vi "GwyddionFileHeader.vi"(8 "error in":errorcluster, 11 "Filename":string) -> (0 "error out":errorcluster)   [LabVIEW 2016]
uses:
  controls/Enum.ctl
  libgwyscan-1.2-labview2015-win32/libgwyscan.lvlib
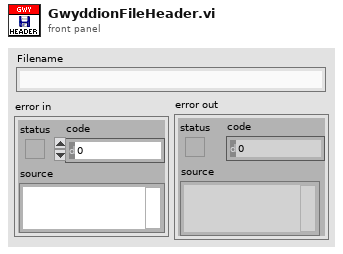
[diagram p1: front panel]
types:
  T1 = typedef "Enum.ctl" = enum16{"Init", "Read", "Write"}
  T2 = cluster{"calibName":string[], "calibParameters":cluster{"Sensitivity":cluster{"Sens X":dbl, "Sens Y":dbl, "Sens Z":dbl}, "Range":cluster{"Range X":dbl, "Range Y":dbl, "Range Z":dbl}, "HV gain":cluster{"HV gain X":dbl, "HV gain Y":dbl, "HV gain Z":dbl}}[], "calibIndex":i32}
  T3 = cluster{"Sensitivity":cluster{"Sens X":dbl, "Sens Y":dbl, "Sens Z":dbl}, "Range":cluster{"Range X":dbl, "Range Y":dbl, "Range Z":dbl}, "HV gain":cluster{"HV gain X":dbl, "HV gain Y":dbl, "HV gain Z":dbl}}[]
  T4 = cluster{"channelsToSaveOut":u8[], "Units":string[], "Saving":cluster{"Fwd":i32[], "Bwd":i32[]}, "x":i32[]}
  T5 = cluster{"Units":string[], "Offsets":dbl[], "Calibrations":dbl[]}
  T6 = cluster{"Sensitivity":cluster{"Sens X":dbl, "Sens Y":dbl, "Sens Z":dbl}, "Range":cluster{"Range X":dbl, "Range Y":dbl, "Range Z":dbl}, "HV gain":cluster{"HV gain X":dbl, "HV gain Y":dbl, "HV gain Z":dbl}}
  T7 = cluster{"Width":dbl, "Height":dbl, "X Offset":dbl, "Y Offset":dbl, "Angle":dbl, "Pixels/Line":u16, "Lines":u16, "Time/Line":dbl, "Scan Rate":dbl}
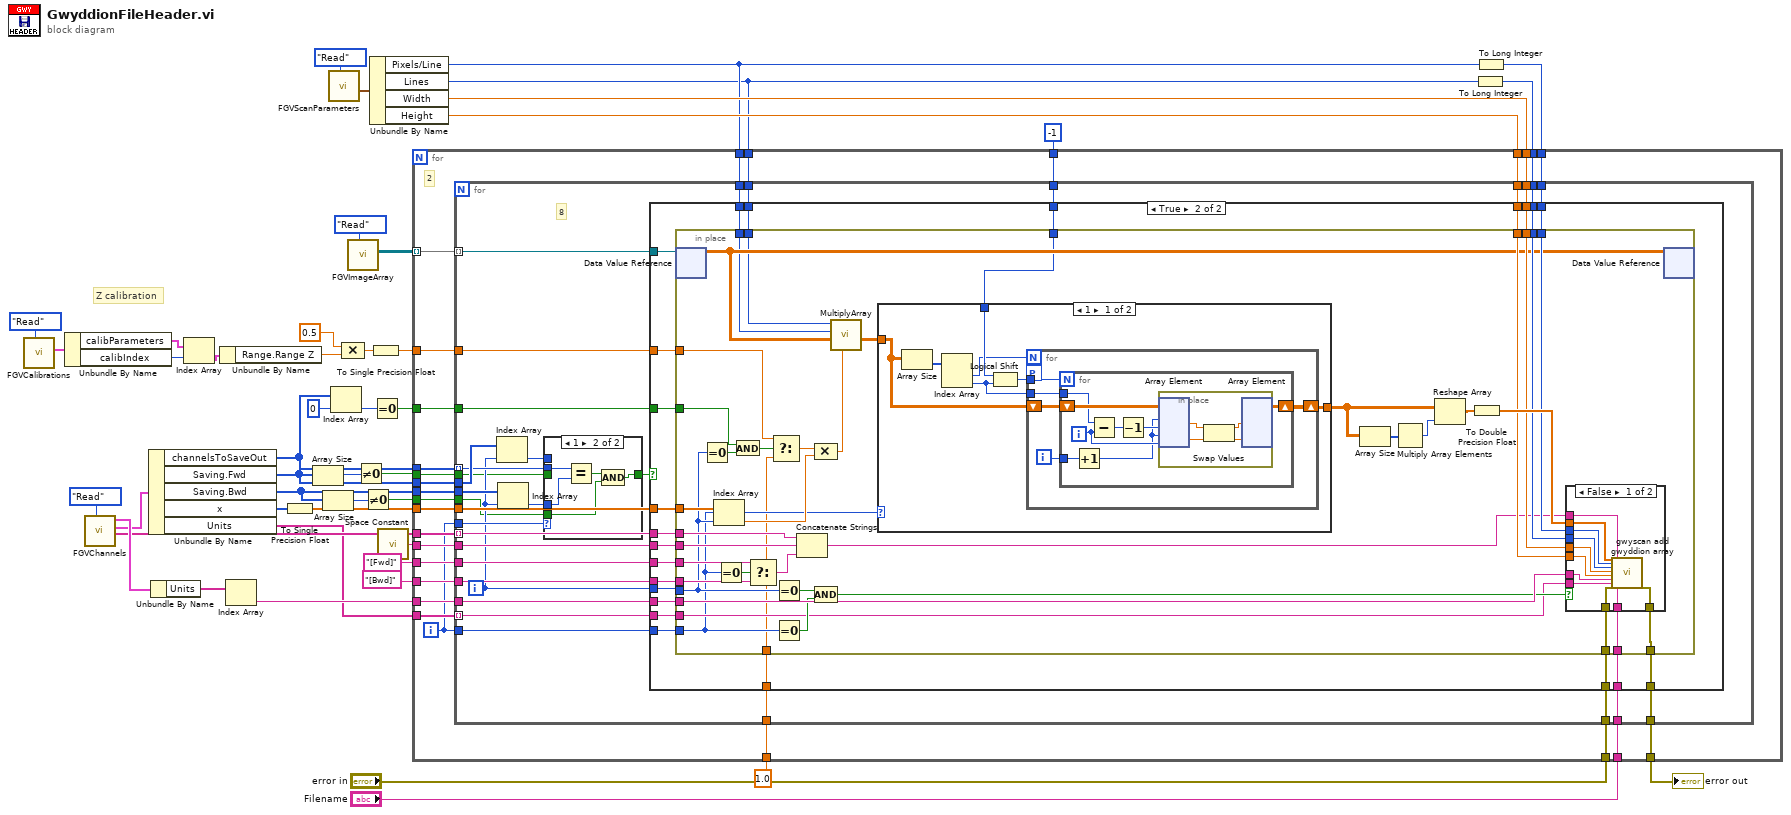
[diagram p0: block diagram]
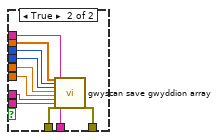
[diagram p3: hidden frame]
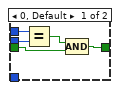
[diagram p5: hidden frame]
diagram:
  # "Z calibration"
  n1 = call "FGVCalibrations.vi"("Enum"=Enum."Read") -> ("calibOut"=w44:T2)  [unwired: 9 in, 1 out]
  n2 = Unbundle By Name(w44) -> ("calibParameters"=w43:T3, "calibIndex"=w42:i32)
  n3 = call "FGVChannels.vi"("Enum"=Enum."Read") -> ("channelsNamesOut"=w26:string[], "SavingChoiceOut"=w12:T4, "XYZ Units/Cal/Offset Out"=w38:T5)  [unwired: 6 in, 2 out]
  n4 = Unbundle By Name(w12) -> ("channelsToSaveOut"=w8:u8[], "Saving.Fwd"=w6:i32[], "Saving.Bwd"=w7:i32[], "x"=w11:i32[], "Units"=w9:string[])
  n5 = Unbundle By Name(w38) -> ("Units"=w35:string[])
  n6 = Index Array(array=w43, index=w42) -> (element=w41:T6)
  n7 = Unbundle By Name(w41) -> ("Range.Range Z"=w40:dbl)
  n8 = Index Array(array=w35) -> (element=w30:string)  [unwired: 1 in]
  n9 = To Single Precision Float(number=w11) -> (single precision float=w10:sgl[])
  n10 = Array Size(array=w6) -> (size(s)=w4:i32)
  n11 = Array Size(array=w7) -> (size(s)=w5:i32)
  n12 = call "FGVScanParameters.vi"("Enum"=Enum."Read") -> ("Scan Parameters Out"=w31:T7)  [unwired: 9 in, 1 out]
  n13 = Index Array(array=w8, index=0) -> (element=w14:u8)
  n14 = Compound Arithmetic op=MULTIPLY(0.5 ("x"), w40) -> (w37:dbl)
  n15 = call "FGVImageArray.vi"("Enum"=Enum."Read") -> ("ImageRefOut"=w34:refnum<data-value>[][])  [unwired: 9 in, 1 out]
  n16 = Not Equal To 0?(x=w4) -> (x != 0?=w3:bool)
  n17 = Not Equal To 0?(x=w5) -> (x != 0?=w2:bool)
  n18 = Unbundle By Name(w31) -> ("Pixels/Line"=w18:u16, "Lines"=w17:u16, "Width"=w20:dbl, "Height"=w19:dbl)
  n19 = To Single Precision Float(number=w37) -> (single precision float=w33:sgl)
  n20 = Equal To 0?(x=w14) -> (x = 0?=w13:bool)
  n21 = call <vilib>:"Space Constant.vi"() -> ("String"=w27:string)
  n22 = To Long Integer(number=w17) -> (32bit integer=w24:i32)
  n23 = To Long Integer(number=w18) -> (32bit integer=w25:i32)
  n24 = for {
    tunnel: w34 -> [w73] mode=indexing
    tunnel: w33 -> [w72]
    tunnel: w30 -> [w71]
    tunnel: "[Bwd]" -> [w70]
    tunnel: "[Fwd]" -> [w69]
    tunnel: w27 -> [w68]
    tunnel: w26 -> [w67]
    tunnel: w9 -> [w66]
    tunnel: w25 -> [w65]
    tunnel: w24 -> [w64]
    tunnel: w20 -> [w63]
    tunnel: w19 -> [w62]
    tunnel: "Filename" -> [w61]
    tunnel: "error in" -> [w60]
    tunnel: [w59] -> w21
    tunnel: w18 -> [w58]
    tunnel: w17 -> [w57]
    tunnel: i16 -1 ("y") -> [w56]
    tunnel: w13 -> [w55]
    tunnel: w10 -> [w54]
    tunnel: w6 -> [w52]
    tunnel: w7 -> [w51]
    tunnel: w8 -> [w53]
    tunnel: w2 -> [w49]
    tunnel: w3 -> [w48]
    tunnel: sgl 1.0 ("f") -> [w47]
    i -> [w50]
    # "2"
    n25 = for {
      tunnel: w73 -> [w105] mode=indexing
      tunnel: w72 -> [w104]
      tunnel: w71 -> [w103]
      tunnel: w70 -> [w102]
      tunnel: w69 -> [w101]
      tunnel: w68 -> [w100]
      tunnel: w67 -> [w99] mode=indexing
      tunnel: w66 -> [w98] mode=indexing
      tunnel: w50 -> [w85]
      tunnel: w65 -> [w97]
      tunnel: w64 -> [w96]
      tunnel: w63 -> [w95]
      tunnel: w62 -> [w94]
      tunnel: w61 -> [w93]
      tunnel: w60 -> [w92]
      tunnel: [w91] -> w59
      tunnel: w58 -> [w90]
      tunnel: w57 -> [w89]
      tunnel: w56 -> [w88]
      tunnel: w55 -> [w87]
      tunnel: w54 -> [w86]
      tunnel: w53 -> [w81] mode=indexing
      tunnel: w52 -> [w83]
      tunnel: w51 -> [w82]
      tunnel: w50 -> [w84]
      tunnel: w49 -> [w75]
      tunnel: w48 -> [w76]
      tunnel: w47 -> [w74]
      i -> [w77]
      # "8"
      n26 = Index Array(array=w83, index=w77) -> (element=w79:i32)
      n27 = Index Array(array=w82, index=w77) -> (element=w78:i32)
      n28 = case shown="1" w84 {
        tunnel: w79 -> [w221 _]
        tunnel: w78 -> [_ w225]
        tunnel: w81 -> [w220 w226]
        tunnel: [w217 w223] -> w80
        tunnel: w76 -> [w219 _]
        tunnel: w75 -> [_ w222]
        frame 0, Default {
          n29 = Equal?(x=w221, y=w220) -> (x = y?=w218:bool)
          n30 = Compound Arithmetic op=AND(w218, w219) -> (w217:bool)
        }
        frame 1 {
          n31 = Equal?(x=w226, y=w225) -> (x = y?=w224:bool)
          n32 = Compound Arithmetic op=AND(w224, w222) -> (w223:bool)
        }
      }
      n33 = case shown="True" w80 {
        tunnel: w105 -> [_ w129]
        tunnel: w104 -> [_ w128]
        tunnel: w103 -> [_ w127]
        tunnel: w102 -> [_ w126]
        tunnel: w101 -> [_ w125]
        tunnel: w100 -> [_ w124]
        tunnel: w99 -> [_ w123]
        tunnel: w98 -> [_ w122]
        tunnel: w97 -> [_ w121]
        tunnel: w96 -> [_ w120]
        tunnel: w95 -> [_ w119]
        tunnel: w94 -> [_ w118]
        tunnel: w93 -> [_ w117]
        tunnel: w92 -> [w106 w116]
        tunnel: [w106 w115] -> w91
        tunnel: w90 -> [_ w114]
        tunnel: w89 -> [_ w113]
        tunnel: w88 -> [_ w112]
        tunnel: w87 -> [_ w111]
        tunnel: w86 -> [_ w110]
        tunnel: w77 -> [_ w109]
        tunnel: w85 -> [_ w108]
        tunnel: w74 -> [_ w107]
        frame False {
        }
        frame True {
          n34 = in-place {
            in-place-border: w128 -> [w146]
            in-place-border: w127 -> [w154]
            in-place-border: w126 -> [w169]
            in-place-border: w125 -> [w168]
            in-place-border: w124 -> [w167]
            in-place-border: w123 -> [w166]
            in-place-border: w122 -> [w136]
            in-place-border: w108 -> [w134]
            in-place-border: w109 -> [w135]
            in-place-border: w121 -> [w158]
            in-place-border: w120 -> [w157]
            in-place-border: w119 -> [w156]
            in-place-border: w118 -> [w155]
            in-place-border: w117 -> [w150]
            in-place-border: w116 -> [w148]
            in-place-border: [w147] -> w115
            in-place-border: w114 -> [w132]
            in-place-border: w113 -> [w131]
            in-place-border: w112 -> [w144]
            in-place-border: w111 -> [w143]
            in-place-border: w110 -> [w140]
            in-place-border: w107 -> [w133]
            n35 = in-place-dvr #1(w129) -> (w145:sgl[][])  [unwired: 1 out]
            n36 = Equal To 0?(x=w135) -> (x = 0?=w142:bool)
            n37 = Index Array(array=w140, index=w135) -> (element=w139:sgl)
            n38 = Equal To 0?(x=w134) -> (x = 0?=w163:bool)
            n39 = And(x=w143, y=w142) -> (x .and. y?=w141:bool)
            n40 = Select(t=w168, s=w163, f=w169) -> (s? t:f=w162:string)
            n41 = Select(t=w146, s=w141, f=w133) -> (s? t:f=w138:sgl)
            n42 = Equal To 0?(x=w135) -> (x = 0?=w152:bool)
            n43 = Equal To 0?(x=w134) -> (x = 0?=w151:bool)
            n44 = Concatenate Strings(w166, w167, w162) -> (w153:string)
            n45 = Compound Arithmetic op=MULTIPLY(w138, w139) -> (w137:sgl)
            n46 = Compound Arithmetic op=AND(w152, w151) -> (w149:bool)
            n47 = call "MultiplyArray.vi"("Calibration"=w137, "DataIn"=w145, "Pixels/Line"=w132, "Lines"=w131) -> ("MultipliedData"=w130:sgl[][])  [unwired: 7 in]
            n48 = case shown="1" w134 {
              tunnel: w130 -> [w198 w216]
              tunnel: [w197 w216] -> w161
              tunnel: w144 -> [w195 _]
              frame 1 {
                n49 = Array Size(array=w198) -> (size(s)=w196:i32[])
                n50 = Index Array(array=w196) -> (element #1=w193:i32, element #2=w192:i32)  [unwired: 2 in]
                n51 = Logical Shift(y=w195, x=w192) -> (x << y=w194:i32)
                n52 = for {
                  N: w193 -> [_]
                  tunnel: w194 -> [w201]
                  shift-right: [w202] -> w197
                  shift-left: w198 -> [w203]
                  workers-P: _ -> [_]
                  tunnel: w192 -> [w199]
                  i -> [w200]
                  n53 = for {
                    N: w201 -> [_]
                    shift-right: [w210] -> w202
                    shift-left: w203 -> [w211]
                    tunnel: w200 -> [w208]
                    tunnel: w199 -> [w204]
                    i -> [w206]
                    n54 = Increment(x=w208) -> (x+1=w205:i32)
                    n55 = Subtract(x=w204, y=w206) -> (x-y=w209:i32)
                    n56 = Decrement(x=w209) -> (x-1=w207:i32)
                    n57 = in-place {
                      n58 = in-place-array #2(w211, w205, w207, w205, w206) -> (w215:sgl, w214:sgl)
                      n59 = Swap Values(12:w215, 14:w214) -> (1:w213:sgl, 3:w212:sgl)  [unwired: 1 in]
                      n60 = in-place-array #2(w213, w212) -> (w210:sgl[][])  [unwired: 4 out]
                    }
                  }
                }
              }
              frame 0, Default {
              }
            }
            n61 = Array Size(array=w161) -> (size(s)=w165:i32[])
            n62 = Multiply Array Elements(1:w165) -> (0:w164:i32)
            n63 = Reshape Array(w161, w164) -> (w160:sgl[])
            n64 = To Double Precision Float(number=w160) -> (double precision float=w159:dbl[])
            n65 = case shown="False" w149 {
              tunnel: w159 -> [w180 w191]
              tunnel: w158 -> [w179 w190]
              tunnel: w157 -> [w178 w189]
              tunnel: w156 -> [w177 w188]
              tunnel: w155 -> [w176 w187]
              tunnel: w154 -> [w175 w186]
              tunnel: w136 -> [w174 w185]
              tunnel: w153 -> [w173 w184]
              tunnel: w150 -> [w172 w183]
              tunnel: w148 -> [w171 w182]
              tunnel: [w170 w181] -> w147
              frame False {
                n66 = call "gwyscan add gwyddion array.vi"("data"=w180, "xres"=w179, "yres"=w178, "xreal"=w177, "yreal"=w176, "xyunit"=w175, "zunit"=w174, "error in (no error)"=w171, "description"=w173, "filename"=w172) -> ("error out"=w170:errorcluster)  [unwired: 11 in, 6 out]
              }
              frame True {
                n67 = call "gwyscan save gwyddion array.vi"("data"=w191, "xres"=w190, "yres"=w189, "xreal"=w188, "yreal"=w187, "xyunit"=w186, "zunit"=w185, "error in (no error)"=w182, "description"=w184, "filename"=w183) -> ("error out"=w181:errorcluster)  [unwired: 11 in, 6 out]
              }
            }
            n68 = in-place-dvr #1(w145) -> ()  [unwired: 2 out]
          }
        }
      }
    }
  }
  "error out" <- w21
